vi "Indent Subsquent Report.vi"(0 "report in":refnum<class "NI_report.lvclass">, 5 "level":i32, 11 "error in (no error)":errorcluster, 12 "MS Office parameters":T1) -> (4 "report out":refnum<class "NI_report.lvclass">, 15 "error out":errorcluster)   [LabVIEW 2020, in "NI_report.lvclass"]
uses:
  NI_report.lvclass
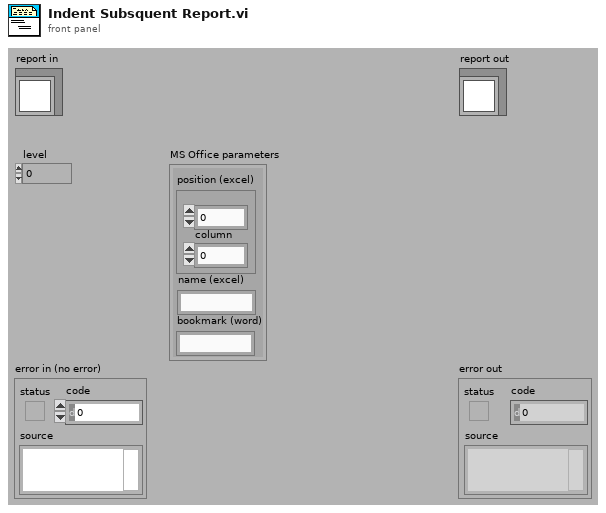
[diagram p1: front panel]
types:
  T1 = cluster{"position (excel)":cluster{"row":i32, "column":i32}, "name (excel)":string, "bookmark (word)":string}
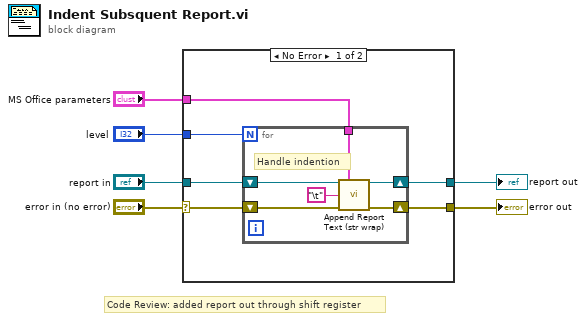
[diagram p0: block diagram]
diagram:
  # "Code Review: added report out through shift register"
  n1 = case shown="No Error" "error in (no error)" {
    selector: "error in (no error)" -> [w8 w20]
    tunnel: [w7 w20] -> w5
    tunnel: [w10 w19] -> w3
    tunnel: "report in" -> [w11 w19]
    tunnel: "MS Office parameters" -> [w12 _]
    tunnel: "level" -> [w9 _]
    frame No Error {
      n2 = for {
        N: w9 -> [_]
        shift-right: [w13] -> w7
        shift-left: w8 -> [w14]
        tunnel: w12 -> [w18]
        shift-right: [w15] -> w10
        shift-left: w11 -> [w16]
        # "Handle indention"
        n3 = call "Append Report Text (str wrap).vi"("report in"=w16, "MS Office parameters"=w18, "text"="\t", "error in (no error)"=w14) -> ("report out"=w15:refnum<class "NI_report.lvclass">, "error out"=w13:errorcluster)  [unwired: 2 in, 8 out]
      }
    }
    frame Error {
    }
  }
  "error out" <- w5
  "report out" <- w3
